vi "Get Data.vi"(8 "error in":errorcluster, 11 "connection ID In":refnum<k5>) -> (0 "error out":errorcluster, 2 "Data":string, 3 "connection ID Out":refnum<k5>)   [LabVIEW 2018, in "Labview Python.lvlib"]
uses:
  Labview Python.lvlib
panel:
  out "Numeric":i32
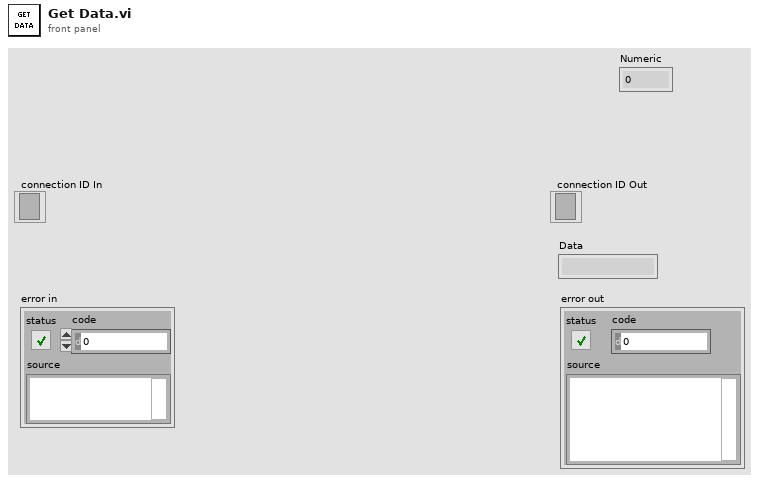
[diagram p1: front panel]
types:
  T1 = enum16{"Standard", "Buffered", "CRLF", "Immediate"}
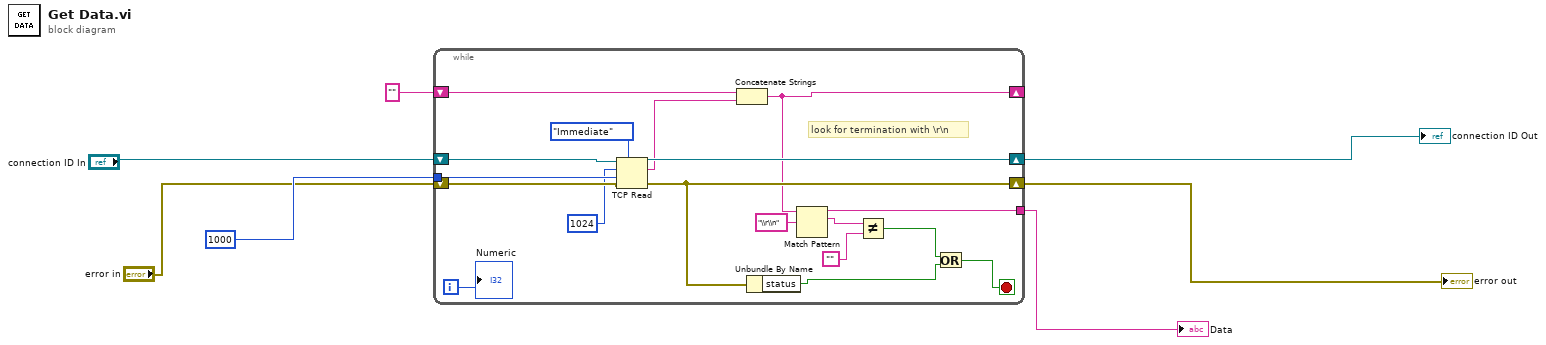
[diagram p0: block diagram]
diagram:
  n1 = while {
    tunnel: 1000 ("timeout ms (25000)") -> [w24]
    shift-right: [w25] -> w6
    shift-left: "connection ID In" -> [w23]
    shift-right: [w13] -> w7
    shift-left: "error in" -> [w22]
    shift-right: [w12] -> _
    shift-left: "" -> [w20]
    tunnel: [w15] -> w1
    i -> [w8]
    stop <- w10 stop-if-true
    # "look for termination with \\r\\n"
    n2 = TCP Read(connection ID=w23, bytes to read=1024, error in (no error)=w22, 7:T1."Immediate" ("mode (standard)"), 9:w24) -> (connection ID out=w25:refnum<k5>, data out=w19:string, error out=w13:errorcluster)
    n3 = Concatenate Strings(w20, w19) -> (w12:string)
    n4 = Unbundle By Name(w13) -> ("status"=w9:bool)
    n5 = Match Pattern(string=w12, regular expression="\\r\\n") -> (before substring=w15:string, match substring=w17:string)  [unwired: 1 in, 2 out]
    n6 = Not Equal?(x=w17, y="") -> (x != y?=w11:bool)
    n7 = Or(x=w11, y=w9) -> (x .or. y?=w10:bool)
    "Numeric" <- w8
  }
  "Data" <- w1
  "connection ID Out" <- w6
  "error out" <- w7
